vi "App - analyze RUS V6.vi"() -> ()   [LabVIEW 2015] (continued)
"radius"=0.0}}, "timestamp(min)"=2417.0666666701436, "timestamp"=timestamp(3493872845 s since 1904-01-01), "Magn Field(T)"=0.0}, {"temperature"=14.354, "lorentzian"={"Amplitude"=0.0, "omega(0)"=0.0, "Gamma"=0.0, "phase"=0.0, "Q"=0.0, "Norm  Ampl"=0.0, "z (inf)"=0.0+0.0i, "4corners"={"z (-pi/2)"=0.0+0.0i, "z(inf)"=0.0+0.0i, "z (pi/2)"=0.0+0.0i, "z center"=0.0+0.0i, "z(0)"=0.0+0.0i, "radius"=0.0}}, "timestamp(min)"=2418.3833333328366, "timestamp"=timestamp(3493872924 s since 1904-01-01), "Magn Field(T)"=0.0}, {"temperature"=14.349, "lorentzian"={"Amplitude"=0.0, "omega(0)"=0.0, "Gamma"=0.0, "phase"=0.0, "Q"=0.0, "Norm  Ampl"=0.0, "z (inf)"=0.0+0.0i, "4corners"={"z (-pi/2)"=0.0+0.0i, "z(inf)"=0.0+0.0i, "z (pi/2)"=0.0+0.0i, "z center"=0.0+0.0i, "z(0)"=0.0+0.0i, "radius"=0.0}}, "timestamp(min)"=2419.7000000029802, "timestamp"=timestamp(3493873003 s since 1904-01-01), "Magn Field(T)"=0.0}, {"temperature"=14.349, "lorentzian"={"Amplitude"=0.0, "omega(0)"=0.0, "Gamma"=0.0, "phase"=0.0, "Q"=0.0, "Norm  Ampl"=0.0, "z (inf)"=0.0+0.0i, "4corners"={"z (-pi/2)"=0.0+0.0i, "z(inf)"=0.0+0.0i, "z (pi/2)"=0.0+0.0i, "z center"=0.0+0.0i, "z(0)"=0.0+0.0i, "radius"=0.0}}, "timestamp(min)"=2421.0333333313465, "timestamp"=timestamp(3493873083 s since 1904-01-01), "Magn Field(T)"=0.0}, {"temperature"=14.346, "lorentzian"={"Amplitude"=0.0, "omega(0)"=0.0, "Gamma"=0.0, "phase"=0.0, "Q"=0.0, "Norm  Ampl"=0.0, "z (inf)"=0.0+0.0i, "4corners"={"z (-pi/2)"=0.0+0.0i, "z(inf)"=0.0+0.0i, "z (pi/2)"=0.0+0.0i, "z center"=0.0+0.0i, "z(0)"=0.0+0.0i, "radius"=0.0}}, "timestamp(min)"=2422.35000000149, "timestamp"=timestamp(3493873162 s since 1904-01-01), "Magn Field(T)"=0.0}, {"temperature"=14.344, "lorentzian"={"Amplitude"=0.0, "omega(0)"=0.0, "Gamma"=0.0, "phase"=0.0, "Q"=0.0, "Norm  Ampl"=0.0, "z (inf)"=0.0+0.0i, "4corners"={"z (-pi/2)"=0.0+0.0i, "z(inf)"=0.0+0.0i, "z (pi/2)"=0.0+0.0i, "z center"=0.0+0.0i, "z(0)"=0.0+0.0i, "radius"=0.0}}, "timestamp(min)"=2423.683333337307, "timestamp"=timestamp(3493873242 s since 1904-01-01), "Magn Field(T)"=0.0}, {"temperature"=14.346, "lorentzian"={"Amplitude"=0.0, "omega(0)"=0.0, "Gamma"=0.0, "phase"=0.0, "Q"=0.0, "Norm  Ampl"=0.0, "z (inf)"=0.0+0.0i, "4corners"={"z (-pi/2)"=0.0+0.0i, "z(inf)"=0.0+0.0i, "z (pi/2)"=0.0+0.0i, "z center"=0.0+0.0i, "z(0)"=0.0+0.0i, "radius"=0.0}}, "timestamp(min)"=2425.0, "timestamp"=timestamp(3493873321 s since 1904-01-01), "Magn Field(T)"=0.0}, {"temperature"=14.346, "lorentzian"={"Amplitude"=0.0, "omega(0)"=0.0, "Gamma"=0.0, "phase"=0.0, "Q"=0.0, "Norm  Ampl"=0.0, "z (inf)"=0.0+0.0i, "4corners"={"z (-pi/2)"=0.0+0.0i, "z(inf)"=0.0+0.0i, "z (pi/2)"=0.0+0.0i, "z center"=0.0+0.0i, "z(0)"=0.0+0.0i, "radius"=0.0}}, "timestamp(min)"=2426.3166666701436, "timestamp"=timestamp(3493873400 s since 1904-01-01), "Magn Field(T)"=0.0}, {"temperature"=14.348, "lorentzian"={"Amplitude"=0.0, "omega(0)"=0.0, "Gamma"=0.0, "phase"=0.0, "Q"=0.0, "Norm  Ampl"=0.0, "z (inf)"=0.0+0.0i, "4corners"={"z (-pi/2)"=0.0+0.0i, "z(inf)"=0.0+0.0i, "z (pi/2)"=0.0+0.0i, "z center"=0.0+0.0i, "z(0)"=0.0+0.0i, "radius"=0.0}}, "timestamp(min)"=2427.64999999851, "timestamp"=timestamp(3493873480 s since 1904-01-01), "Magn Field(T)"=0.0}, {"temperature"=14.353, "lorentzian"={"Amplitude"=0.0, "omega(0)"=0.0, "Gamma"=0.0, "phase"=0.0, "Q"=0.0, "Norm  Ampl"=0.0, "z (inf)"=0.0+0.0i, "4corners"={"z (-pi/2)"=0.0+0.0i, "z(inf)"=0.0+0.0i, "z (pi/2)"=0.0+0.0i, "z center"=0.0+0.0i, "z(0)"=0.0+0.0i, "radius"=0.0}}, "timestamp(min)"=2428.9666666686535, "timestamp"=timestamp(3493873559 s since 1904-01-01), "Magn Field(T)"=0.0}, {"temperature"=14.355, "lorentzian"={"Amplitude"=0.0, "omega(0)"=0.0, "Gamma"=0.0, "phase"=0.0, "Q"=0.0, "Norm  Ampl"=0.0, "z (inf)"=0.0+0.0i, "4corners"={"z (-pi/2)"=0.0+0.0i, "z(inf)"=0.0+0.0i, "z (pi/2)"=0.0+0.0i, "z center"=0.0+0.0i, "z(0)"=0.0+0.0i, "radius"=0.0}}, "timestamp(min)"=2430.2833333313465, "timestamp"=timestamp(3493873638 s since 1904-01-01), "Magn Field(T)"=0.0}, {"temperature"=14.349, "lorentzian"={"Amplitude"=0.0, "omega(0)"=0.0, "Gamma"=0.0, "phase"=0.0, "Q"=0.0, "Norm  Ampl"=0.0, "z (inf)"=0.0+0.0i, "4corners"={"z (-pi/2)"=0.0+0.0i, "z(inf)"=0.0+0.0i, "z (pi/2)"=0.0+0.0i, "z center"=0.0+0.0i, "z(0)"=0.0+0.0i, "radius"=0.0}}, "timestamp(min)"=2431.6166666671634, "timestamp"=timestamp(3493873718 s since 1904-01-01), "Magn Field(T)"=0.0}, {"temperature"=14.351, "lorentzian"={"Amplitude"=0.0, "omega(0)"=0.0, "Gamma"=0.0, "phase"=0.0, "Q"=0.0, "Norm  Ampl"=0.0, "z (inf)"=0.0+0.0i, "4corners"={"z (-pi/2)"=0.0+0.0i, "z(inf)"=0.0+0.0i, "z (pi/2)"=0.0+0.0i, "z center"=0.0+0.0i, "z(0)"=0.0+0.0i, "radius"=0.0}}, "timestamp(min)"=2432.933333337307, "timestamp"=timestamp(3493873797 s since 1904-01-01), "Magn Field(T)"=0.0}, {"temperature"=14.35, "lorentzian"={"Amplitude"=0.0, "omega(0)"=0.0, "Gamma"=0.0, "phase"=0.0, "Q"=0.0, "Norm  Ampl"=0.0, "z (inf)"=0.0+0.0i, "4corners"={"z (-pi/2)"=0.0+0.0i, "z(inf)"=0.0+0.0i, "z (pi/2)"=0.0+0.0i, "z center"=0.0+0.0i, "z(0)"=0.0+0.0i, "radius"=0.0}}, "timestamp(min)"=2434.2666666656733, "timestamp"=timestamp(3493873877 s since 1904-01-01), "Magn Field(T)"=0.0}, {"temperature"=14.347, "lorentzian"={"Amplitude"=0.0, "omega(0)"=0.0, "Gamma"=0.0, "phase"=0.0, "Q"=0.0, "Norm  Ampl"=0.0, "z (inf)"=0.0+0.0i, "4corners"={"z (-pi/2)"=0.0+0.0i, "z(inf)"=0.0+0.0i, "z (pi/2)"=0.0+0.0i, "z center"=0.0+0.0i, "z(0)"=0.0+0.0i, "radius"=0.0}}, "timestamp(min)"=2435.583333335817, "timestamp"=timestamp(3493873956 s since 1904-01-01), "Magn Field(T)"=0.0}, {"temperature"=14.35, "lorentzian"={"Amplitude"=0.0, "omega(0)"=0.0, "Gamma"=0.0, "phase"=0.0, "Q"=0.0, "Norm  Ampl"=0.0, "z (inf)"=0.0+0.0i, "4corners"={"z (-pi/2)"=0.0+0.0i, "z(inf)"=0.0+0.0i, "z (pi/2)"=0.0+0.0i, "z center"=0.0+0.0i, "z(0)"=0.0+0.0i, "radius"=0.0}}, "timestamp(min)"=2436.89999999851, "timestamp"=timestamp(3493874035 s since 1904-01-01), "Magn Field(T)"=0.0}, {"temperature"=14.349, "lorentzian"={"Amplitude"=0.0, "omega(0)"=0.0, "Gamma"=0.0, "phase"=0.0, "Q"=0.0, "Norm  Ampl"=0.0, "z (inf)"=0.0+0.0i, "4corners"={"z (-pi/2)"=0.0+0.0i, "z(inf)"=0.0+0.0i, "z (pi/2)"=0.0+0.0i, "z center"=0.0+0.0i, "z(0)"=0.0+0.0i, "radius"=0.0}}, "timestamp(min)"=2438.2333333343267, "timestamp"=timestamp(3493874115 s since 1904-01-01), "Magn Field(T)"=0.0}, {"temperature"=14.35, "lorentzian"={"Amplitude"=0.0, "omega(0)"=0.0, "Gamma"=0.0, "phase"=0.0, "Q"=0.0, "Norm  Ampl"=0.0, "z (inf)"=0.0+0.0i, "4corners"={"z (-pi/2)"=0.0+0.0i, "z(inf)"=0.0+0.0i, "z (pi/2)"=0.0+0.0i, "z center"=0.0+0.0i, "z(0)"=0.0+0.0i, "radius"=0.0}}, "timestamp(min)"=2439.5500000044703, "timestamp"=timestamp(3493874194 s since 1904-01-01), "Magn Field(T)"=0.0}, {"temperature"=14.351, "lorentzian"={"Amplitude"=0.0, "omega(0)"=0.0, "Gamma"=0.0, "phase"=0.0, "Q"=0.0, "Norm  Ampl"=0.0, "z (inf)"=0.0+0.0i, "4corners"={"z (-pi/2)"=0.0+0.0i, "z(inf)"=0.0+0.0i, "z (pi/2)"=0.0+0.0i, "z center"=0.0+0.0i, "z(0)"=0.0+0.0i, "radius"=0.0}}, "timestamp(min)"=2440.8666666671634, "timestamp"=timestamp(3493874273 s since 1904-01-01), "Magn Field(T)"=0.0}, {"temperature"=14.351, "lorentzian"={"Amplitude"=0.0, "omega(0)"=0.0, "Gamma"=0.0, "phase"=0.0, "Q"=0.0, "Norm  Ampl"=0.0, "z (inf)"=0.0+0.0i, "4corners"={"z (-pi/2)"=0.0+0.0i, "z(inf)"=0.0+0.0i, "z (pi/2)"=0.0+0.0i, "z center"=0.0+0.0i, "z(0)"=0.0+0.0i, "radius"=0.0}}, "timestamp(min)"=2442.2000000029802, "timestamp"=timestamp(3493874353 s since 1904-01-01), "Magn Field(T)"=0.0}, {"temperature"=14.352, "lorentzian"={"Amplitude"=0.0, "omega(0)"=0.0, "Gamma"=0.0, "phase"=0.0, "Q"=0.0, "Norm  Ampl"=0.0, "z (inf)"=0.0+0.0i, "4corners"={"z (-pi/2)"=0.0+0.0i, "z(inf)"=0.0+0.0i, "z (pi/2)"=0.0+0.0i, "z center"=0.0+0.0i, "z(0)"=0.0+0.0i, "radius"=0.0}}, "timestamp(min)"=2443.5166666656733, "timestamp"=timestamp(3493874432 s since 1904-01-01), "Magn Field(T)"=0.0}, {"temperature"=14.351, "lorentzian"={"Amplitude"=0.0, "omega(0)"=0.0, "Gamma"=0.0, "phase"=0.0, "Q"=0.0, "Norm  Ampl"=0.0, "z (inf)"=0.0+0.0i, "4corners"={"z (-pi/2)"=0.0+0.0i, "z(inf)"=0.0+0.0i, "z (pi/2)"=0.0+0.0i, "z center"=0.0+0.0i, "z(0)"=0.0+0.0i, "radius"=0.0}}, "timestamp(min)"=2444.85000000149, "timestamp"=timestamp(3493874512 s since 1904-01-01), "Magn Field(T)"=0.0}, {"temperature"=14.35, "lorentzian"={"Amplitude"=0.0, "omega(0)"=0.0, "Gamma"=0.0, "phase"=0.0, "Q"=0.0, "Norm  Ampl"=0.0, "z (inf)"=0.0+0.0i, "4corners"={"z (-pi/2)"=0.0+0.0i, "z(inf)"=0.0+0.0i, "z (pi/2)"=0.0+0.0i, "z center"=0.0+0.0i, "z(0)"=0.0+0.0i, "radius"=0.0}}, "timestamp(min)"=2446.166666664183, "timestamp"=timestamp(3493874591 s since 1904-01-01), "Magn Field(T)"=0.0}, {"temperature"=14.353, "lorentzian"={"Amplitude"=0.0, "omega(0)"=0.0, "Gamma"=0.0, "phase"=0.0, "Q"=0.0, "Norm  Ampl"=0.0, "z (inf)"=0.0+0.0i, "4corners"={"z (-pi/2)"=0.0+0.0i, "z(inf)"=0.0+0.0i, "z (pi/2)"=0.0+0.0i, "z center"=0.0+0.0i, "z(0)"=0.0+0.0i, "radius"=0.0}}, "timestamp(min)"=2447.4833333343267, "timestamp"=timestamp(3493874670 s since 1904-01-01), "Magn Field(T)"=0.0}, {"temperature"=14.354, "lorentzian"={"Amplitude"=0.0, "omega(0)"=0.0, "Gamma"=0.0, "phase"=0.0, "Q"=0.0, "Norm  Ampl"=0.0, "z (inf)"=0.0+0.0i, "4corners"={"z (-pi/2)"=0.0+0.0i, "z(inf)"=0.0+0.0i, "z (pi/2)"=0.0+0.0i, "z center"=0.0+0.0i, "z(0)"=0.0+0.0i, "radius"=0.0}}, "timestamp(min)"=2448.8166666701436, "timestamp"=timestamp(3493874750 s since 1904-01-01), "Magn Field(T)"=0.0}, {"temperature"=14.356, "lorentzian"={"Amplitude"=0.0, "omega(0)"=0.0, "Gamma"=0.0, "phase"=0.0, "Q"=0.0, "Norm  Ampl"=0.0, "z (inf)"=0.0+0.0i, "4corners"={"z (-pi/2)"=0.0+0.0i, "z(inf)"=0.0+0.0i, "z (pi/2)"=0.0+0.0i, "z center"=0.0+0.0i, "z(0)"=0.0+0.0i, "radius"=0.0}}, "timestamp(min)"=2450.1333333328366, "timestamp"=timestamp(3493874829 s since 1904-01-01), "Magn Field(T)"=0.0}, {"temperature"=14.359, "lorentzian"={"Amplitude"=0.0, "omega(0)"=0.0, "Gamma"=0.0, "phase"=0.0, "Q"=0.0, "Norm  Ampl"=0.0, "z (inf)"=0.0+0.0i, "4corners"={"z (-pi/2)"=0.0+0.0i, "z(inf)"=0.0+0.0i, "z (pi/2)"=0.0+0.0i, "z center"=0.0+0.0i, "z(0)"=0.0+0.0i, "radius"=0.0}}, "timestamp(min)"=2451.4666666686535, "timestamp"=timestamp(3493874909 s since 1904-01-01), "Magn Field(T)"=0.0}, {"temperature"=14.361, "lorentzian"={"Amplitude"=0.0, "omega(0)"=0.0, "Gamma"=0.0, "phase"=0.0, "Q"=0.0, "Norm  Ampl"=0.0, "z (inf)"=0.0+0.0i, "4corners"={"z (-pi/2)"=0.0+0.0i, "z(inf)"=0.0+0.0i, "z (pi/2)"=0.0+0.0i, "z center"=0.0+0.0i, "z(0)"=0.0+0.0i, "radius"=0.0}}, "timestamp(min)"=2452.7833333313465, "timestamp"=timestamp(3493874988 s since 1904-01-01), "Magn Field(T)"=0.0}, {"temperature"=14.36, "lorentzian"={"Amplitude"=0.0, "omega(0)"=0.0, "Gamma"=0.0, "phase"=0.0, "Q"=0.0, "Norm  Ampl"=0.0, "z (inf)"=0.0+0.0i, "4corners"={"z (-pi/2)"=0.0+0.0i, "z(inf)"=0.0+0.0i, "z (pi/2)"=0.0+0.0i, "z center"=0.0+0.0i, "z(0)"=0.0+0.0i, "radius"=0.0}}, "timestamp(min)"=2454.10000000149, "timestamp"=timestamp(3493875067 s since 1904-01-01), "Magn Field(T)"=0.0}, {"temperature"=14.364, "lorentzian"={"Amplitude"=0.0, "omega(0)"=0.0, "Gamma"=0.0, "phase"=0.0, "Q"=0.0, "Norm  Ampl"=0.0, "z (inf)"=0.0+0.0i, "4corners"={"z (-pi/2)"=0.0+0.0i, "z(inf)"=0.0+0.0i, "z (pi/2)"=0.0+0.0i, "z center"=0.0+0.0i, "z(0)"=0.0+0.0i, "radius"=0.0}}, "timestamp(min)"=2455.433333337307, "timestamp"=timestamp(3493875147 s since 1904-01-01), "Magn Field(T)"=0.0}, {"temperature"=14.363, "lorentzian"={"Amplitude"=0.0, "omega(0)"=0.0, "Gamma"=0.0, "phase"=0.0, "Q"=0.0, "Norm  Ampl"=0.0, "z (inf)"=0.0+0.0i, "4corners"={"z (-pi/2)"=0.0+0.0i, "z(inf)"=0.0+0.0i, "z (pi/2)"=0.0+0.0i, "z center"=0.0+0.0i, "z(0)"=0.0+0.0i, "radius"=0.0}}, "timestamp(min)"=2456.75, "timestamp"=timestamp(3493875226 s since 1904-01-01), "Magn Field(T)"=0.0}, {"temperature"=14.368, "lorentzian"={"Amplitude"=0.0, "omega(0)"=0.0, "Gamma"=0.0, "phase"=0.0, "Q"=0.0, "Norm  Ampl"=0.0, "z (inf)"=0.0+0.0i, "4corners"={"z (-pi/2)"=0.0+0.0i, "z(inf)"=0.0+0.0i, "z (pi/2)"=0.0+0.0i, "z center"=0.0+0.0i, "z(0)"=0.0+0.0i, "radius"=0.0}}, "timestamp(min)"=2458.0666666701436, "timestamp"=timestamp(3493875305 s since 1904-01-01), "Magn Field(T)"=0.0}, {"temperature"=14.367, "lorentzian"={"Amplitude"=0.0, "omega(0)"=0.0, "Gamma"=0.0, "phase"=0.0, "Q"=0.0, "Norm  Ampl"=0.0, "z (inf)"=0.0+0.0i, "4corners"={"z (-pi/2)"=0.0+0.0i, "z(inf)"=0.0+0.0i, "z (pi/2)"=0.0+0.0i, "z center"=0.0+0.0i, "z(0)"=0.0+0.0i, "radius"=0.0}}, "timestamp(min)"=2459.39999999851, "timestamp"=timestamp(3493875385 s since 1904-01-01), "Magn Field(T)"=0.0}, {"temperature"=14.368, "lorentzian"={"Amplitude"=0.0, "omega(0)"=0.0, "Gamma"=0.0, "phase"=0.0, "Q"=0.0, "Norm  Ampl"=0.0, "z (inf)"=0.0+0.0i, "4corners"={"z (-pi/2)"=0.0+0.0i, "z(inf)"=0.0+0.0i, "z (pi/2)"=0.0+0.0i, "z center"=0.0+0.0i, "z(0)"=0.0+0.0i, "radius"=0.0}}, "timestamp(min)"=2460.7166666686535, "timestamp"=timestamp(3493875464 s since 1904-01-01), "Magn Field(T)"=0.0}, {"temperature"=14.368, "lorentzian"={"Amplitude"=0.0, "omega(0)"=0.0, "Gamma"=0.0, "phase"=0.0, "Q"=0.0, "Norm  Ampl"=0.0, "z (inf)"=0.0+0.0i, "4corners"={"z (-pi/2)"=0.0+0.0i, "z(inf)"=0.0+0.0i, "z (pi/2)"=0.0+0.0i, "z center"=0.0+0.0i, "z(0)"=0.0+0.0i, "radius"=0.0}}, "timestamp(min)"=2462.0500000044703, "timestamp"=timestamp(3493875544 s since 1904-01-01), "Magn Field(T)"=0.0}, {"temperature"=14.366, "lorentzian"={"Amplitude"=0.0, "omega(0)"=0.0, "Gamma"=0.0, "phase"=0.0, "Q"=0.0, "Norm  Ampl"=0.0, "z (inf)"=0.0+0.0i, "4corners"={"z (-pi/2)"=0.0+0.0i, "z(inf)"=0.0+0.0i, "z (pi/2)"=0.0+0.0i, "z center"=0.0+0.0i, "z(0)"=0.0+0.0i, "radius"=0.0}}, "timestamp(min)"=2463.3666666671634, "timestamp"=timestamp(3493875623 s since 1904-01-01), "Magn Field(T)"=0.0}, {"temperature"=14.369, "lorentzian"={"Amplitude"=0.0, "omega(0)"=0.0, "Gamma"=0.0, "phase"=0.0, "Q"=0.0, "Norm  Ampl"=0.0, "z (inf)"=0.0+0.0i, "4corners"={"z (-pi/2)"=0.0+0.0i, "z(inf)"=0.0+0.0i, "z (pi/2)"=0.0+0.0i, "z center"=0.0+0.0i, "z(0)"=0.0+0.0i, "radius"=0.0}}, "timestamp(min)"=2464.683333337307, "timestamp"=timestamp(3493875702 s since 1904-01-01), "Magn Field(T)"=0.0}, {"temperature"=14.369, "lorentzian"={"Amplitude"=0.0, "omega(0)"=0.0, "Gamma"=0.0, "phase"=0.0, "Q"=0.0, "Norm  Ampl"=0.0, "z (inf)"=0.0+0.0i, "4corners"={"z (-pi/2)"=0.0+0.0i, "z(inf)"=0.0+0.0i, "z (pi/2)"=0.0+0.0i, "z center"=0.0+0.0i, "z(0)"=0.0+0.0i, "radius"=0.0}}, "timestamp(min)"=2466.0166666656733, "timestamp"=timestamp(3493875782 s since 1904-01-01), "Magn Field(T)"=0.0}, {"temperature"=14.371, "lorentzian"={"Amplitude"=0.0, "omega(0)"=0.0, "Gamma"=0.0, "phase"=0.0, "Q"=0.0, "Norm  Ampl"=0.0, "z (inf)"=0.0+0.0i, "4corners"={"z (-pi/2)"=0.0+0.0i, "z(inf)"=0.0+0.0i, "z (pi/2)"=0.0+0.0i, "z center"=0.0+0.0i, "z(0)"=0.0+0.0i, "radius"=0.0}}, "timestamp(min)"=2467.333333335817, "timestamp"=timestamp(3493875861 s since 1904-01-01), "Magn Field(T)"=0.0}, {"temperature"=14.377, "lorentzian"={"Amplitude"=0.0, "omega(0)"=0.0, "Gamma"=0.0, "phase"=0.0, "Q"=0.0, "Norm  Ampl"=0.0, "z (inf)"=0.0+0.0i, "4corners"={"z (-pi/2)"=0.0+0.0i, "z(inf)"=0.0+0.0i, "z (pi/2)"=0.0+0.0i, "z center"=0.0+0.0i, "z(0)"=0.0+0.0i, "radius"=0.0}}, "timestamp(min)"=2468.64999999851, "timestamp"=timestamp(3493875940 s since 1904-01-01), "Magn Field(T)"=0.0}, {"temperature"=14.377, "lorentzian"={"Amplitude"=0.0, "omega(0)"=0.0, "Gamma"=0.0, "phase"=0.0, "Q"=0.0, "Norm  Ampl"=0.0, "z (inf)"=0.0+0.0i, "4corners"={"z (-pi/2)"=0.0+0.0i, "z(inf)"=0.0+0.0i, "z (pi/2)"=0.0+0.0i, "z center"=0.0+0.0i, "z(0)"=0.0+0.0i, "radius"=0.0}}, "timestamp(min)"=2469.9833333343267, "timestamp"=timestamp(3493876020 s since 1904-01-01), "Magn Field(T)"=0.0}, {"temperature"=14.374, "lorentzian"={"Amplitude"=0.0, "omega(0)"=0.0, "Gamma"=0.0, "phase"=0.0, "Q"=0.0, "Norm  Ampl"=0.0, "z (inf)"=0.0+0.0i, "4corners"={"z (-pi/2)"=0.0+0.0i, "z(inf)"=0.0+0.0i, "z (pi/2)"=0.0+0.0i, "z center"=0.0+0.0i, "z(0)"=0.0+0.0i, "radius"=0.0}}, "timestamp(min)"=2471.3000000044703, "timestamp"=timestamp(3493876099 s since 1904-01-01), "Magn Field(T)"=0.0}, {"temperature"=14.374, "lorentzian"={"Amplitude"=0.0, "omega(0)"=0.0, "Gamma"=0.0, "phase"=0.0, "Q"=0.0, "Norm  Ampl"=0.0, "z (inf)"=0.0+0.0i, "4corners"={"z (-pi/2)"=0.0+0.0i, "z(inf)"=0.0+0.0i, "z (pi/2)"=0.0+0.0i, "z center"=0.0+0.0i, "z(0)"=0.0+0.0i, "radius"=0.0}}, "timestamp(min)"=2472.6333333328366, "timestamp"=timestamp(3493876179 s since 1904-01-01), "Magn Field(T)"=0.0}, {"temperature"=14.376, "lorentzian"={"Amplitude"=0.0, "omega(0)"=0.0, "Gamma"=0.0, "phase"=0.0, "Q"=0.0, "Norm  Ampl"=0.0, "z (inf)"=0.0+0.0i, "4corners"={"z (-pi/2)"=0.0+0.0i, "z(inf)"=0.0+0.0i, "z (pi/2)"=0.0+0.0i, "z center"=0.0+0.0i, "z(0)"=0.0+0.0i, "radius"=0.0}}, "timestamp(min)"=2473.9500000029802, "timestamp"=timestamp(3493876258 s since 1904-01-01), "Magn Field(T)"=0.0}, {"temperature"=14.375, "lorentzian"={"Amplitude"=0.0, "omega(0)"=0.0, "Gamma"=0.0, "phase"=0.0, "Q"=0.0, "Norm  Ampl"=0.0, "z (inf)"=0.0+0.0i, "4corners"={"z (-pi/2)"=0.0+0.0i, "z(inf)"=0.0+0.0i, "z (pi/2)"=0.0+0.0i, "z center"=0.0+0.0i, "z(0)"=0.0+0.0i, "radius"=0.0}}, "timestamp(min)"=2475.2666666656733, "timestamp"=timestamp(3493876337 s since 1904-01-01), "Magn Field(T)"=0.0}, {"temperature"=14.379, "lorentzian"={"Amplitude"=0.0, "omega(0)"=0.0, "Gamma"=0.0, "phase"=0.0, "Q"=0.0, "Norm  Ampl"=0.0, "z (inf)"=0.0+0.0i, "4corners"={"z (-pi/2)"=0.0+0.0i, "z(inf)"=0.0+0.0i, "z (pi/2)"=0.0+0.0i, "z center"=0.0+0.0i, "z(0)"=0.0+0.0i, "radius"=0.0}}, "timestamp(min)"=2476.60000000149, "timestamp"=timestamp(3493876417 s since 1904-01-01), "Magn Field(T)"=0.0}, {"temperature"=14.38, "lorentzian"={"Amplitude"=0.0, "omega(0)"=0.0, "Gamma"=0.0, "phase"=0.0, "Q"=0.0, "Norm  Ampl"=0.0, "z (inf)"=0.0+0.0i, "4corners"={"z (-pi/2)"=0.0+0.0i, "z(inf)"=0.0+0.0i, "z (pi/2)"=0.0+0.0i, "z center"=0.0+0.0i, "z(0)"=0.0+0.0i, "radius"=0.0}}, "timestamp(min)"=2477.916666664183, "timestamp"=timestamp(3493876496 s since 1904-01-01), "Magn Field(T)"=0.0}, {"temperature"=14.384, "lorentzian"={"Amplitude"=0.0, "omega(0)"=0.0, "Gamma"=0.0, "phase"=0.0, "Q"=0.0, "Norm  Ampl"=0.0, "z (inf)"=0.0+0.0i, "4corners"={"z (-pi/2)"=0.0+0.0i, "z(inf)"=0.0+0.0i, "z (pi/2)"=0.0+0.0i, "z center"=0.0+0.0i, "z(0)"=0.0+0.0i, "radius"=0.0}}, "timestamp(min)"=2479.25, "timestamp"=timestamp(3493876576 s since 1904-01-01), "Magn Field(T)"=0.0}, {"temperature"=14.382, "lorentzian"={"Amplitude"=0.0, "omega(0)"=0.0, "Gamma"=0.0, "phase"=0.0, "Q"=0.0, "Norm  Ampl"=0.0, "z (inf)"=0.0+0.0i, "4corners"={"z (-pi/2)"=0.0+0.0i, "z(inf)"=0.0+0.0i, "z (pi/2)"=0.0+0.0i, "z center"=0.0+0.0i, "z(0)"=0.0+0.0i, "radius"=0.0}}, "timestamp(min)"=2480.5666666701436, "timestamp"=timestamp(3493876655 s since 1904-01-01), "Magn Field(T)"=0.0}, {"temperature"=14.383, "lorentzian"={"Amplitude"=0.0, "omega(0)"=0.0, "Gamma"=0.0, "phase"=0.0, "Q"=0.0, "Norm  Ampl"=0.0, "z (inf)"=0.0+0.0i, "4corners"={"z (-pi/2)"=0.0+0.0i, "z(inf)"=0.0+0.0i, "z (pi/2)"=0.0+0.0i, "z center"=0.0+0.0i, "z(0)"=0.0+0.0i, "radius"=0.0}}, "timestamp(min)"=2481.8833333328366, "timestamp"=timestamp(3493876734 s since 1904-01-01), "Magn Field(T)"=0.0}, {"temperature"=14.382, "lorentzian"={"Amplitude"=0.0, "omega(0)"=0.0, "Gamma"=0.0, "phase"=0.0, "Q"=0.0, "Norm  Ampl"=0.0, "z (inf)"=0.0+0.0i, "4corners"={"z (-pi/2)"=0.0+0.0i, "z(inf)"=0.0+0.0i, "z (pi/2)"=0.0+0.0i, "z center"=0.0+0.0i, "z(0)"=0.0+0.0i, "radius"=0.0}}, "timestamp(min)"=2483.2166666686535, "timestamp"=timestamp(3493876814 s since 1904-01-01), "Magn Field(T)"=0.0}, {"temperature"=14.381, "lorentzian"={"Amplitude"=0.0, "omega(0)"=0.0, "Gamma"=0.0, "phase"=0.0, "Q"=0.0, "Norm  Ampl"=0.0, "z (inf)"=0.0+0.0i, "4corners"={"z (-pi/2)"=0.0+0.0i, "z(inf)"=0.0+0.0i, "z (pi/2)"=0.0+0.0i, "z center"=0.0+0.0i, "z(0)"=0.0+0.0i, "radius"=0.0}}, "timestamp(min)"=2484.5333333313465, "timestamp"=timestamp(3493876893 s since 1904-01-01), "Magn Field(T)"=0.0}, {"temperature"=14.386, "lorentzian"={"Amplitude"=0.0, "omega(0)"=0.0, "Gamma"=0.0, "phase"=0.0, "Q"=0.0, "Norm  Ampl"=0.0, "z (inf)"=0.0+0.0i, "4corners"={"z (-pi/2)"=0.0+0.0i, "z(inf)"=0.0+0.0i, "z (pi/2)"=0.0+0.0i, "z center"=0.0+0.0i, "z(0)"=0.0+0.0i, "radius"=0.0}}, "timestamp(min)"=2485.85000000149, "timestamp"=timestamp(3493876972 s since 1904-01-01), "Magn Field(T)"=0.0}, {"temperature"=14.389, "lorentzian"={"Amplitude"=0.0, "omega(0)"=0.0, "Gamma"=0.0, "phase"=0.0, "Q"=0.0, "Norm  Ampl"=0.0, "z (inf)"=0.0+0.0i, "4corners"={"z (-pi/2)"=0.0+0.0i, "z(inf)"=0.0+0.0i, "z (pi/2)"=0.0+0.0i, "z center"=0.0+0.0i, "z(0)"=0.0+0.0i, "radius"=0.0}}, "timestamp(min)"=2487.183333337307, "timestamp"=timestamp(3493877052 s since 1904-01-01), "Magn Field(T)"=0.0}, {"temperature"=14.392, "lorentzian"={"Amplitude"=0.0, "omega(0)"=0.0, "Gamma"=0.0, "phase"=0.0, "Q"=0.0, "Norm  Ampl"=0.0, "z (inf)"=0.0+0.0i, "4corners"={"z (-pi/2)"=0.0+0.0i, "z(inf)"=0.0+0.0i, "z (pi/2)"=0.0+0.0i, "z center"=0.0+0.0i, "z(0)"=0.0+0.0i, "radius"=0.0}}, "timestamp(min)"=2488.5, "timestamp"=timestamp(3493877131 s since 1904-01-01), "Magn Field(T)"=0.0}, {"temperature"=14.395, "lorentzian"={"Amplitude"=0.0, "omega(0)"=0.0, "Gamma"=0.0, "phase"=0.0, "Q"=0.0, "Norm  Ampl"=0.0, "z (inf)"=0.0+0.0i, "4corners"={"z (-pi/2)"=0.0+0.0i, "z(inf)"=0.0+0.0i, "z (pi/2)"=0.0+0.0i, "z center"=0.0+0.0i, "z(0)"=0.0+0.0i, "radius"=0.0}}, "timestamp(min)"=2489.833333335817, "timestamp"=timestamp(3493877211 s since 1904-01-01), "Magn Field(T)"=0.0}, {"temperature"=14.397, "lorentzian"={"Amplitude"=0.0, "omega(0)"=0.0, "Gamma"=0.0, "phase"=0.0, "Q"=0.0, "Norm  Ampl"=0.0, "z (inf)"=0.0+0.0i, "4corners"={"z (-pi/2)"=0.0+0.0i, "z(inf)"=0.0+0.0i, "z (pi/2)"=0.0+0.0i, "z center"=0.0+0.0i, "z(0)"=0.0+0.0i, "radius"=0.0}}, "timestamp(min)"=2491.14999999851, "timestamp"=timestamp(3493877290 s since 1904-01-01), "Magn Field(T)"=0.0}, {"temperature"=14.399, "lorentzian"={"Amplitude"=0.0, "omega(0)"=0.0, "Gamma"=0.0, "phase"=0.0, "Q"=0.0, "Norm  Ampl"=0.0, "z (inf)"=0.0+0.0i, "4corners"={"z (-pi/2)"=0.0+0.0i, "z(inf)"=0.0+0.0i, "z (pi/2)"=0.0+0.0i, "z center"=0.0+0.0i, "z(0)"=0.0+0.0i, "radius"=0.0}}, "timestamp(min)"=2492.4666666686535, "timestamp"=timestamp(3493877369 s since 1904-01-01), "Magn Field(T)"=0.0}, {"temperature"=14.4, "lorentzian"={"Amplitude"=0.0, "omega(0)"=0.0, "Gamma"=0.0, "phase"=0.0, "Q"=0.0, "Norm  Ampl"=0.0, "z (inf)"=0.0+0.0i, "4corners"={"z (-pi/2)"=0.0+0.0i, "z(inf)"=0.0+0.0i, "z (pi/2)"=0.0+0.0i, "z center"=0.0+0.0i, "z(0)"=0.0+0.0i, "radius"=0.0}}, "timestamp(min)"=2493.8000000044703, "timestamp"=timestamp(3493877449 s since 1904-01-01), "Magn Field(T)"=0.0}, {"temperature"=14.404, "lorentzian"={"Amplitude"=0.0, "omega(0)"=0.0, "Gamma"=0.0, "phase"=0.0, "Q"=0.0, "Norm  Ampl"=0.0, "z (inf)"=0.0+0.0i, "4corners"={"z (-pi/2)"=0.0+0.0i, "z(inf)"=0.0+0.0i, "z (pi/2)"=0.0+0.0i, "z center"=0.0+0.0i, "z(0)"=0.0+0.0i, "radius"=0.0}}, "timestamp(min)"=2495.1166666671634, "timestamp"=timestamp(3493877528 s since 1904-01-01), "Magn Field(T)"=0.0}, {"temperature"=14.405, "lorentzian"={"Amplitude"=0.0, "omega(0)"=0.0, "Gamma"=0.0, "phase"=0.0, "Q"=0.0, "Norm  Ampl"=0.0, "z (inf)"=0.0+0.0i, "4corners"={"z (-pi/2)"=0.0+0.0i, "z(inf)"=0.0+0.0i, "z (pi/2)"=0.0+0.0i, "z center"=0.0+0.0i, "z(0)"=0.0+0.0i, "radius"=0.0}}, "timestamp(min)"=2496.4500000029802, "timestamp"=timestamp(3493877608 s since 1904-01-01), "Magn Field(T)"=0.0}, {"temperature"=14.407, "lorentzian"={"Amplitude"=0.0, "omega(0)"=0.0, "Gamma"=0.0, "phase"=0.0, "Q"=0.0, "Norm  Ampl"=0.0, "z (inf)"=0.0+0.0i, "4corners"={"z (-pi/2)"=0.0+0.0i, "z(inf)"=0.0+0.0i, "z (pi/2)"=0.0+0.0i, "z center"=0.0+0.0i, "z(0)"=0.0+0.0i, "radius"=0.0}}, "timestamp(min)"=2497.7666666656733, "timestamp"=timestamp(3493877687 s since 1904-01-01), "Magn Field(T)"=0.0}, {"temperature"=14.411, "lorentzian"={"Amplitude"=0.0, "omega(0)"=0.0, "Gamma"=0.0, "phase"=0.0, "Q"=0.0, "Norm  Ampl"=0.0, "z (inf)"=0.0+0.0i, "4corners"={"z (-pi/2)"=0.0+0.0i, "z(inf)"=0.0+0.0i, "z (pi/2)"=0.0+0.0i, "z center"=0.0+0.0i, "z(0)"=0.0+0.0i, "radius"=0.0}}, "timestamp(min)"=2499.083333335817, "timestamp"=timestamp(3493877766 s since 1904-01-01), "Magn Field(T)"=0.0}, {"temperature"=14.416, "lorentzian"={"Amplitude"=0.0, "omega(0)"=0.0, "Gamma"=0.0, "phase"=0.0, "Q"=0.0, "Norm  Ampl"=0.0, "z (inf)"=0.0+0.0i, "4corners"={"z (-pi/2)"=0.0+0.0i, "z(inf)"=0.0+0.0i, "z (pi/2)"=0.0+0.0i, "z center"=0.0+0.0i, "z(0)"=0.0+0.0i, "radius"=0.0}}, "timestamp(min)"=2500.416666664183, "timestamp"=timestamp(3493877846 s since 1904-01-01), "Magn Field(T)"=0.0}, {"temperature"=14.42, "lorentzian"={"Amplitude"=0.0, "omega(0)"=0.0, "Gamma"=0.0, "phase"=0.0, "Q"=0.0, "Norm  Ampl"=0.0, "z (inf)"=0.0+0.0i, "4corners"={"z (-pi/2)"=0.0+0.0i, "z(inf)"=0.0+0.0i, "z (pi/2)"=0.0+0.0i, "z center"=0.0+0.0i, "z(0)"=0.0+0.0i, "radius"=0.0}}, "timestamp(min)"=2501.7333333343267, "timestamp"=timestamp(3493877925 s since 1904-01-01), "Magn Field(T)"=0.0}, {"temperature"=14.42, "lorentzian"={"Amplitude"=0.0, "omega(0)"=0.0, "Gamma"=0.0, "phase"=0.0, "Q"=0.0, "Norm  Ampl"=0.0, "z (inf)"=0.0+0.0i, "4corners"={"z (-pi/2)"=0.0+0.0i, "z(inf)"=0.0+0.0i, "z (pi/2)"=0.0+0.0i, "z center"=0.0+0.0i, "z(0)"=0.0+0.0i, "radius"=0.0}}, "timestamp(min)"=2503.0500000044703, "timestamp"=timestamp(3493878004 s since 1904-01-01), "Magn Field(T)"=0.0}, {"temperature"=14.42, "lorentzian"={"Amplitude"=0.0, "omega(0)"=0.0, "Gamma"=0.0, "phase"=0.0, "Q"=0.0, "Norm  Ampl"=0.0, "z (inf)"=0.0+0.0i, "4corners"={"z (-pi/2)"=0.0+0.0i, "z(inf)"=0.0+0.0i, "z (pi/2)"=0.0+0.0i, "z center"=0.0+0.0i, "z(0)"=0.0+0.0i, "radius"=0.0}}, "timestamp(min)"=2504.3833333328366, "timestamp"=timestamp(3493878084 s since 1904-01-01), "Magn Field(T)"=0.0}, {"temperature"=14.42, "lorentzian"={"Amplitude"=0.0, "omega(0)"=0.0, "Gamma"=0.0, "phase"=0.0, "Q"=0.0, "Norm  Ampl"=0.0, "z (inf)"=0.0+0.0i, "4corners"={"z (-pi/2)"=0.0+0.0i, "z(inf)"=0.0+0.0i, "z (pi/2)"=0.0+0.0i, "z center"=0.0+0.0i, "z(0)"=0.0+0.0i, "radius"=0.0}}, "timestamp(min)"=2505.7000000029802, "timestamp"=timestamp(3493878163 s since 1904-01-01), "Magn Field(T)"=0.0}, {"temperature"=14.426, "lorentzian"={"Amplitude"=0.0, "omega(0)"=0.0, "Gamma"=0.0, "phase"=0.0, "Q"=0.0, "Norm  Ampl"=0.0, "z (inf)"=0.0+0.0i, "4corners"={"z (-pi/2)"=0.0+0.0i, "z(inf)"=0.0+0.0i, "z (pi/2)"=0.0+0.0i, "z center"=0.0+0.0i, "z(0)"=0.0+0.0i, "radius"=0.0}}, "timestamp(min)"=2507.0333333313465, "timestamp"=timestamp(3493878243 s since 1904-01-01), "Magn Field(T)"=0.0}, {"temperature"=14.427, "lorentzian"={"Amplitude"=0.0, "omega(0)"=0.0, "Gamma"=0.0, "phase"=0.0, "Q"=0.0, "Norm  Ampl"=0.0, "z (inf)"=0.0+0.0i, "4corners"={"z (-pi/2)"=0.0+0.0i, "z(inf)"=0.0+0.0i, "z (pi/2)"=0.0+0.0i, "z center"=0.0+0.0i, "z(0)"=0.0+0.0i, "radius"=0.0}}, "timestamp(min)"=2508.35000000149, "timestamp"=timestamp(3493878322 s since 1904-01-01), "Magn Field(T)"=0.0}, {"temperature"=14.431, "lorentzian"={"Amplitude"=0.0, "omega(0)"=0.0, "Gamma"=0.0, "phase"=0.0, "Q"=0.0, "Norm  Ampl"=0.0, "z (inf)"=0.0+0.0i, "4corners"={"z (-pi/2)"=0.0+0.0i, "z(inf)"=0.0+0.0i, "z (pi/2)"=0.0+0.0i, "z center"=0.0+0.0i, "z(0)"=0.0+0.0i, "radius"=0.0}}, "timestamp(min)"=2509.666666664183, "timestamp"=timestamp(3493878401 s since 1904-01-01), "Magn Field(T)"=0.0}, {"temperature"=14.43, "lorentzian"={"Amplitude"=0.0, "omega(0)"=0.0, "Gamma"=0.0, "phase"=0.0, "Q"=0.0, "Norm  Ampl"=0.0, "z (inf)"=0.0+0.0i, "4corners"={"z (-pi/2)"=0.0+0.0i, "z(inf)"=0.0+0.0i, "z (pi/2)"=0.0+0.0i, "z center"=0.0+0.0i, "z(0)"=0.0+0.0i, "radius"=0.0}}, "timestamp(min)"=2511.0, "timestamp"=timestamp(3493878481 s since 1904-01-01), "Magn Field(T)"=0.0}, {"temperature"=14.431, "lorentzian"={"Amplitude"=0.0, "omega(0)"=0.0, "Gamma"=0.0, "phase"=0.0, "Q"=0.0, "Norm  Ampl"=0.0, "z (inf)"=0.0+0.0i, "4corners"={"z (-pi/2)"=0.0+0.0i, "z(inf)"=0.0+0.0i, "z (pi/2)"=0.0+0.0i, "z center"=0.0+0.0i, "z(0)"=0.0+0.0i, "radius"=0.0}}, "timestamp(min)"=2512.3166666701436, "timestamp"=timestamp(3493878560 s since 1904-01-01), "Magn Field(T)"=0.0}, {"temperature"=14.433, "lorentzian"={"Amplitude"=0.0, "omega(0)"=0.0, "Gamma"=0.0, "phase"=0.0, "Q"=0.0, "Norm  Ampl"=0.0, "z (inf)"=0.0+0.0i, "4corners"={"z (-pi/2)"=0.0+0.0i, "z(inf)"=0.0+0.0i, "z (pi/2)"=0.0+0.0i, "z center"=0.0+0.0i, "z(0)"=0.0+0.0i, "radius"=0.0}}, "timestamp(min)"=2513.64999999851, "timestamp"=timestamp(3493878640 s since 1904-01-01), "Magn Field(T)"=0.0}, {"temperature"=14.438, "lorentzian"={"Amplitude"=0.0, "omega(0)"=0.0, "Gamma"=0.0, "phase"=0.0, "Q"=0.0, "Norm  Ampl"=0.0, "z (inf)"=0.0+0.0i, "4corners"={"z (-pi/2)"=0.0+0.0i, "z(inf)"=0.0+0.0i, "z (pi/2)"=0.0+0.0i, "z center"=0.0+0.0i, "z(0)"=0.0+0.0i, "radius"=0.0}}, "timestamp(min)"=2514.9666666686535, "timestamp"=timestamp(3493878719 s since 1904-01-01), "Magn Field(T)"=0.0}, {"temperature"=14.434, "lorentzian"={"Amplitude"=0.0, "omega(0)"=0.0, "Gamma"=0.0, "phase"=0.0, "Q"=0.0, "Norm  Ampl"=0.0, "z (inf)"=0.0+0.0i, "4corners"={"z (-pi/2)"=0.0+0.0i, "z(inf)"=0.0+0.0i, "z (pi/2)"=0.0+0.0i, "z center"=0.0+0.0i, "z(0)"=0.0+0.0i, "radius"=0.0}}, "timestamp(min)"=2516.2833333313465, "timestamp"=timestamp(3493878798 s since 1904-01-01), "Magn Field(T)"=0.0}, {"temperature"=14.438, "lorentzian"={"Amplitude"=0.0, "omega(0)"=0.0, "Gamma"=0.0, "phase"=0.0, "Q"=0.0, "Norm  Ampl"=0.0, "z (inf)"=0.0+0.0i, "4corners"={"z (-pi/2)"=0.0+0.0i, "z(inf)"=0.0+0.0i, "z (pi/2)"=0.0+0.0i, "z center"=0.0+0.0i, "z(0)"=0.0+0.0i, "radius"=0.0}}, "timestamp(min)"=2517.6166666671634, "timestamp"=timestamp(3493878878 s since 1904-01-01), "Magn Field(T)"=0.0}, {"temperature"=14.441, "lorentzian"={"Amplitude"=0.0, "omega(0)"=0.0, "Gamma"=0.0, "phase"=0.0, "Q"=0.0, "Norm  Ampl"=0.0, "z (inf)"=0.0+0.0i, "4corners"={"z (-pi/2)"=0.0+0.0i, "z(inf)"=0.0+0.0i, "z (pi/2)"=0.0+0.0i, "z center"=0.0+0.0i, "z(0)"=0.0+0.0i, "radius"=0.0}}, "timestamp(min)"=2518.933333337307, "timestamp"=timestamp(3493878957 s since 1904-01-01), "Magn Field(T)"=0.0}, {"temperature"=14.441, "lorentzian"={"Amplitude"=0.0, "omega(0)"=0.0, "Gamma"=0.0, "phase"=0.0, "Q"=0.0, "Norm  Ampl"=0.0, "z (inf)"=0.0+0.0i, "4corners"={"z (-pi/2)"=0.0+0.0i, "z(inf)"=0.0+0.0i, "z (pi/2)"=0.0+0.0i, "z center"=0.0+0.0i, "z(0)"=0.0+0.0i, "radius"=0.0}}, "timestamp(min)"=2520.25, "timestamp"=timestamp(3493879036 s since 1904-01-01), "Magn Field(T)"=0.0}, {"temperature"=14.444, "lorentzian"={"Amplitude"=0.0, "omega(0)"=0.0, "Gamma"=0.0, "phase"=0.0, "Q"=0.0, "Norm  Ampl"=0.0, "z (inf)"=0.0+0.0i, "4corners"={"z (-pi/2)"=0.0+0.0i, "z(inf)"=0.0+0.0i, "z (pi/2)"=0.0+0.0i, "z center"=0.0+0.0i, "z(0)"=0.0+0.0i, "radius"=0.0}}, "timestamp(min)"=2521.583333335817, "timestamp"=timestamp(3493879116 s since 1904-01-01), "Magn Field(T)"=0.0}, {"temperature"=14.44, "lorentzian"={"Amplitude"=0.0, "omega(0)"=0.0, "Gamma"=0.0, "phase"=0.0, "Q"=0.0, "Norm  Ampl"=0.0, "z (inf)"=0.0+0.0i, "4corners"={"z (-pi/2)"=0.0+0.0i, "z(inf)"=0.0+0.0i, "z (pi/2)"=0.0+0.0i, "z center"=0.0+0.0i, "z(0)"=0.0+0.0i, "radius"=0.0}}, "timestamp(min)"=2522.89999999851, "timestamp"=timestamp(3493879195 s since 1904-01-01), "Magn Field(T)"=0.0}, {"temperature"=14.446, "lorentzian"={"Amplitude"=0.0, "omega(0)"=0.0, "Gamma"=0.0, "phase"=0.0, "Q"=0.0, "Norm  Ampl"=0.0, "z (inf)"=0.0+0.0i, "4corners"={"z (-pi/2)"=0.0+0.0i, "z(inf)"=0.0+0.0i, "z (pi/2)"=0.0+0.0i, "z center"=0.0+0.0i, "z(0)"=0.0+0.0i, "radius"=0.0}}, "timestamp(min)"=2524.2333333343267, "timestamp"=timestamp(3493879275 s since 1904-01-01), "Magn Field(T)"=0.0}, {"temperature"=14.449, "lorentzian"={"Amplitude"=0.0, "omega(0)"=0.0, "Gamma"=0.0, "phase"=0.0, "Q"=0.0, "Norm  Ampl"=0.0, "z (inf)"=0.0+0.0i, "4corners"={"z (-pi/2)"=0.0+0.0i, "z(inf)"=0.0+0.0i, "z (pi/2)"=0.0+0.0i, "z center"=0.0+0.0i, "z(0)"=0.0+0.0i, "radius"=0.0}}, "timestamp(min)"=2525.5500000044703, "timestamp"=timestamp(3493879354 s since 1904-01-01), "Magn Field(T)"=0.0}, {"temperature"=14.447, "lorentzian"={"Amplitude"=0.0, "omega(0)"=0.0, "Gamma"=0.0, "phase"=0.0, "Q"=0.0, "Norm  Ampl"=0.0, "z (inf)"=0.0+0.0i, "4corners"={"z (-pi/2)"=0.0+0.0i, "z(inf)"=0.0+0.0i, "z (pi/2)"=0.0+0.0i, "z center"=0.0+0.0i, "z(0)"=0.0+0.0i, "radius"=0.0}}, "timestamp(min)"=2526.8666666671634, "timestamp"=timestamp(3493879433 s since 1904-01-01), "Magn Field(T)"=0.0}, {"temperature"=14.448, "lorentzian"={"Amplitude"=0.0, "omega(0)"=0.0, "Gamma"=0.0, "phase"=0.0, "Q"=0.0, "Norm  Ampl"=0.0, "z (inf)"=0.0+0.0i, "4corners"={"z (-pi/2)"=0.0+0.0i, "z(inf)"=0.0+0.0i, "z (pi/2)"=0.0+0.0i, "z center"=0.0+0.0i, "z(0)"=0.0+0.0i, "radius"=0.0}}, "timestamp(min)"=2528.2000000029802, "timestamp"=timestamp(3493879513 s since 1904-01-01), "Magn Field(T)"=0.0}, {"temperature"=14.453, "lorentzian"={"Amplitude"=0.0, "omega(0)"=0.0, "Gamma"=0.0, "phase"=0.0, "Q"=0.0, "Norm  Ampl"=0.0, "z (inf)"=0.0+0.0i, "4corners"={"z (-pi/2)"=0.0+0.0i, "z(inf)"=0.0+0.0i, "z (pi/2)"=0.0+0.0i, "z center"=0.0+0.0i, "z(0)"=0.0+0.0i, "radius"=0.0}}, "timestamp(min)"=2529.5166666656733, "timestamp"=timestamp(3493879592 s since 1904-01-01), "Magn Field(T)"=0.0}, {"temperature"=14.45, "lorentzian"={"Amplitude"=0.0, "omega(0)"=0.0, "Gamma"=0.0, "phase"=0.0, "Q"=0.0, "Norm  Ampl"=0.0, "z (inf)"=0.0+0.0i, "4corners"={"z (-pi/2)"=0.0+0.0i, "z(inf)"=0.0+0.0i, "z (pi/2)"=0.0+0.0i, "z center"=0.0+0.0i, "z(0)"=0.0+0.0i, "radius"=0.0}}, "timestamp(min)"=2530.833333335817, "timestamp"=timestamp(3493879671 s since 1904-01-01), "Magn Field(T)"=0.0}, {"temperature"=14.451, "lorentzian"={"Amplitude"=0.0, "omega(0)"=0.0, "Gamma"=0.0, "phase"=0.0, "Q"=0.0, "Norm  Ampl"=0.0, "z (inf)"=0.0+0.0i, "4corners"={"z (-pi/2)"=0.0+0.0i, "z(inf)"=0.0+0.0i, "z (pi/2)"=0.0+0.0i, "z center"=0.0+0.0i, "z(0)"=0.0+0.0i, "radius"=0.0}}, "timestamp(min)"=2532.166666664183, "timestamp"=timestamp(3493879751 s since 1904-01-01), "Magn Field(T)"=0.0}, {"temperature"=14.449, "lorentzian"={"Amplitude"=0.0, "omega(0)"=0.0, "Gamma"=0.0, "phase"=0.0, "Q"=0.0, "Norm  Ampl"=0.0, "z (inf)"=0.0+0.0i, "4corners"={"z (-pi/2)"=0.0+0.0i, "z(inf)"=0.0+0.0i, "z (pi/2)"=0.0+0.0i, "z center"=0.0+0.0i, "z(0)"=0.0+0.0i, "radius"=0.0}}, "timestamp(min)"=2533.4833333343267, "timestamp"=timestamp(3493879830 s since 1904-01-01), "Magn Field(T)"=0.0}, {"temperature"=14.45, "lorentzian"={"Amplitude"=0.0, "omega(0)"=0.0, "Gamma"=0.0, "phase"=0.0, "Q"=0.0, "Norm  Ampl"=0.0, "z (inf)"=0.0+0.0i, "4corners"={"z (-pi/2)"=0.0+0.0i, "z(inf)"=0.0+0.0i, "z (pi/2)"=0.0+0.0i, "z center"=0.0+0.0i, "z(0)"=0.0+0.0i, "radius"=0.0}}, "timestamp(min)"=2534.8166666701436, "timestamp"=timestamp(3493879910 s since 1904-01-01), "Magn Field(T)"=0.0}, {"temperature"=14.453, "lorentzian"={"Amplitude"=0.0, "omega(0)"=0.0, "Gamma"=0.0, "phase"=0.0, "Q"=0.0, "Norm  Ampl"=0.0, "z (inf)"=0.0+0.0i, "4corners"={"z (-pi/2)"=0.0+0.0i, "z(inf)"=0.0+0.0i, "z (pi/2)"=0.0+0.0i, "z center"=0.0+0.0i, "z(0)"=0.0+0.0i, "radius"=0.0}}, "timestamp(min)"=2536.1333333328366, "timestamp"=timestamp(3493879989 s since 1904-01-01), "Magn Field(T)"=0.0}, {"temperature"=14.455, "lorentzian"={"Amplitude"=0.0, "omega(0)"=0.0, "Gamma"=0.0, "phase"=0.0, "Q"=0.0, "Norm  Ampl"=0.0, "z (inf)"=0.0+0.0i, "4corners"={"z (-pi/2)"=0.0+0.0i, "z(inf)"=0.0+0.0i, "z (pi/2)"=0.0+0.0i, "z center"=0.0+0.0i, "z(0)"=0.0+0.0i, "radius"=0.0}}, "timestamp(min)"=2537.4500000029802, "timestamp"=timestamp(3493880068 s since 1904-01-01), "Magn Field(T)"=0.0}, {"temperature"=14.456, "lorentzian"={"Amplitude"=0.0, "omega(0)"=0.0, "Gamma"=0.0, "phase"=0.0, "Q"=0.0, "Norm  Ampl"=0.0, "z (inf)"=0.0+0.0i, "4corners"={"z (-pi/2)"=0.0+0.0i, "z(inf)"=0.0+0.0i, "z (pi/2)"=0.0+0.0i, "z center"=0.0+0.0i, "z(0)"=0.0+0.0i, "radius"=0.0}}, "timestamp(min)"=2538.7833333313465, "timestamp"=timestamp(3493880148 s since 1904-01-01), "Magn Field(T)"=0.0}, {"temperature"=14.457, "lorentzian"={"Amplitude"=0.0, "omega(0)"=0.0, "Gamma"=0.0, "phase"=0.0, "Q"=0.0, "Norm  Ampl"=0.0, "z (inf)"=0.0+0.0i, "4corners"={"z (-pi/2)"=0.0+0.0i, "z(inf)"=0.0+0.0i, "z (pi/2)"=0.0+0.0i, "z center"=0.0+0.0i, "z(0)"=0.0+0.0i, "radius"=0.0}}, "timestamp(min)"=2540.10000000149, "timestamp"=timestamp(3493880227 s since 1904-01-01), "Magn Field(T)"=0.0}, {"temperature"=14.458, "lorentzian"={"Amplitude"=0.0, "omega(0)"=0.0, "Gamma"=0.0, "phase"=0.0, "Q"=0.0, "Norm  Ampl"=0.0, "z (inf)"=0.0+0.0i, "4corners"={"z (-pi/2)"=0.0+0.0i, "z(inf)"=0.0+0.0i, "z (pi/2)"=0.0+0.0i, "z center"=0.0+0.0i, "z(0)"=0.0+0.0i, "radius"=0.0}}, "timestamp(min)"=2541.433333337307, "timestamp"=timestamp(3493880307 s since 1904-01-01), "Magn Field(T)"=0.0}, {"temperature"=14.455, "lorentzian"={"Amplitude"=0.0, "omega(0)"=0.0, "Gamma"=0.0, "phase"=0.0, "Q"=0.0, "Norm  Ampl"=0.0, "z (inf)"=0.0+0.0i, "4corners"={"z (-pi/2)"=0.0+0.0i, "z(inf)"=0.0+0.0i, "z (pi/2)"=0.0+0.0i, "z center"=0.0+0.0i, "z(0)"=0.0+0.0i, "radius"=0.0}}, "timestamp(min)"=2542.75, "timestamp"=timestamp(3493880386 s since 1904-01-01), "Magn Field(T)"=0.0}, {"temperature"=14.459, "lorentzian"={"Amplitude"=0.0, "omega(0)"=0.0, "Gamma"=0.0, "phase"=0.0, "Q"=0.0, "Norm  Ampl"=0.0, "z (inf)"=0.0+0.0i, "4corners"={"z (-pi/2)"=0.0+0.0i, "z(inf)"=0.0+0.0i, "z (pi/2)"=0.0+0.0i, "z center"=0.0+0.0i, "z(0)"=0.0+0.0i, "radius"=0.0}}, "timestamp(min)"=2544.0666666701436, "timestamp"=timestamp(3493880465 s since 1904-01-01), "Magn Field(T)"=0.0}, {"temperature"=14.46, "lorentzian"={"Amplitude"=0.0, "omega(0)"=0.0, "Gamma"=0.0, "phase"=0.0, "Q"=0.0, "Norm  Ampl"=0.0, "z (inf)"=0.0+0.0i, "4corners"={"z (-pi/2)"=0.0+0.0i, "z(inf)"=0.0+0.0i, "z (pi/2)"=0.0+0.0i, "z center"=0.0+0.0i, "z(0)"=0.0+0.0i, "radius"=0.0}}, "timestamp(min)"=2545.39999999851, "timestamp"=timestamp(3493880545 s since 1904-01-01), "Magn Field(T)"=0.0}, {"temperature"=14.459, "lorentzian"={"Amplitude"=0.0, "omega(0)"=0.0, "Gamma"=0.0, "phase"=0.0, "Q"=0.0, "Norm  Ampl"=0.0, "z (inf)"=0.0+0.0i, "4corners"={"z (-pi/2)"=0.0+0.0i, "z(inf)"=0.0+0.0i, "z (pi/2)"=0.0+0.0i, "z center"=0.0+0.0i, "z(0)"=0.0+0.0i, "radius"=0.0}}, "timestamp(min)"=2546.7166666686535, "timestamp"=timestamp(3493880624 s since 1904-01-01), "Magn Field(T)"=0.0}, {"temperature"=14.461, "lorentzian"={"Amplitude"=0.0, "omega(0)"=0.0, "Gamma"=0.0, "phase"=0.0, "Q"=0.0, "Norm  Ampl"=0.0, "z (inf)"=0.0+0.0i, "4corners"={"z (-pi/2)"=0.0+0.0i, "z(inf)"=0.0+0.0i, "z (pi/2)"=0.0+0.0i, "z center"=0.0+0.0i, "z(0)"=0.0+0.0i, "radius"=0.0}}, "timestamp(min)"=2548.0333333313465, "timestamp"=timestamp(3493880703 s since 1904-01-01), "Magn Field(T)"=0.0}, {"temperature"=14.465, "lorentzian"={"Amplitude"=0.0, "omega(0)"=0.0, "Gamma"=0.0, "phase"=0.0, "Q"=0.0, "Norm  Ampl"=0.0, "z (inf)"=0.0+0.0i, "4corners"={"z (-pi/2)"=0.0+0.0i, "z(inf)"=0.0+0.0i, "z (pi/2)"=0.0+0.0i, "z center"=0.0+0.0i, "z(0)"=0.0+0.0i, "radius"=0.0}}, "timestamp(min)"=2549.3666666671634, "timestamp"=timestamp(3493880783 s since 1904-01-01), "Magn Field(T)"=0.0}, {"temperature"=14.467, "lorentzian"={"Amplitude"=0.0, "omega(0)"=0.0, "Gamma"=0.0, "phase"=0.0, "Q"=0.0, "Norm  Ampl"=0.0, "z (inf)"=0.0+0.0i, "4corners"={"z (-pi/2)"=0.0+0.0i, "z(inf)"=0.0+0.0i, "z (pi/2)"=0.0+0.0i, "z center"=0.0+0.0i, "z(0)"=0.0+0.0i, "radius"=0.0}}, "timestamp(min)"=2550.683333337307, "timestamp"=timestamp(3493880862 s since 1904-01-01), "Magn Field(T)"=0.0}, {"temperature"=14.467, "lorentzian"={"Amplitude"=0.0, "omega(0)"=0.0, "Gamma"=0.0, "phase"=0.0, "Q"=0.0, "Norm  Ampl"=0.0, "z (inf)"=0.0+0.0i, "4corners"={"z (-pi/2)"=0.0+0.0i, "z(inf)"=0.0+0.0i, "z (pi/2)"=0.0+0.0i, "z center"=0.0+0.0i, "z(0)"=0.0+0.0i, "radius"=0.0}}, "timestamp(min)"=2552.0166666656733, "timestamp"=timestamp(3493880942 s since 1904-01-01), "Magn Field(T)"=0.0}, {"temperature"=14.469, "lorentzian"={"Amplitude"=0.0, "omega(0)"=0.0, "Gamma"=0.0, "phase"=0.0, "Q"=0.0, "Norm  Ampl"=0.0, "z (inf)"=0.0+0.0i, "4corners"={"z (-pi/2)"=0.0+0.0i, "z(inf)"=0.0+0.0i, "z (pi/2)"=0.0+0.0i, "z center"=0.0+0.0i, "z(0)"=0.0+0.0i, "radius"=0.0}}, "timestamp(min)"=2553.333333335817, "timestamp"=timestamp(3493881021 s since 1904-01-01), "Magn Field(T)"=0.0}, {"temperature"=14.467, "lorentzian"={"Amplitude"=0.0, "omega(0)"=0.0, "Gamma"=0.0, "phase"=0.0, "Q"=0.0, "Norm  Ampl"=0.0, "z (inf)"=0.0+0.0i, "4corners"={"z (-pi/2)"=0.0+0.0i, "z(inf)"=0.0+0.0i, "z (pi/2)"=0.0+0.0i, "z center"=0.0+0.0i, "z(0)"=0.0+0.0i, "radius"=0.0}}, "timestamp(min)"=2554.64999999851, "timestamp"=timestamp(3493881100 s since 1904-01-01), "Magn Field(T)"=0.0}, {"temperature"=14.467, "lorentzian"={"Amplitude"=0.0, "omega(0)"=0.0, "Gamma"=0.0, 
